vi "VisionDetect.vi"(9 "Name":string="Numeric") -> ()   [LabVIEW 2020]
uses:
  <vilib>/Rock Robotics/Network Tables/NT Write Number.vi
  <vilib>/Rock Robotics/Network Tables/NT Read Number.vi
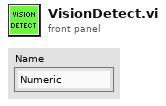
[diagram p1: front panel]
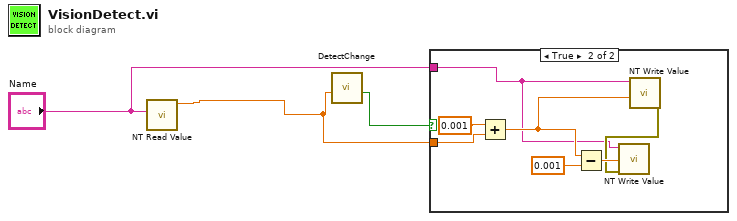
[diagram p0: block diagram]
diagram:
  n1 = call-poly <vilib>:"NT Read Value.vi"("Name"="Name") -> ("Numeric"=w2:dbl)  [unwired: 9 in, 1 out]
  n2 = call "DetectChange.vi"("Numeric"=w2) -> ("Boolean"=w3:bool)  [unwired: 10 in]
  n3 = case shown="True" w3 {
    tunnel: w2 -> [_ w9]
    tunnel: "Name" -> [_ w4]
    frame False {
    }
    frame True {
      n4 = Add(x=0.001, y=w9) -> (x+y=w6:dbl)
      n5 = Subtract(x=w6, y=0.001) -> (x-y=w7:dbl)
      n6 = call-poly <vilib>:"NT Write Value.vi"("Numeric"=w6, "Name"=w4) -> ("error out"=w5:errorcluster)  [unwired: 9 in]
      n7 = call-poly <vilib>:"NT Write Value.vi"("error in"=w5, "Numeric"=w7, "Name"=w4) -> ()  [unwired: 8 in, 1 out]
    }
  }
